vi "FestoCPX.Station.TowerHorn.Fglb.vi"(7 "Action (get)":T1=enum."get", 8 "error in":errorcluster, 10 "Period [s]":dbl) -> (0 "error out":errorcluster, 2 "Done?":bool)   [LabVIEW 2016]
uses:
  FestoCPX.Station.TowerHorn.Fglb.Action.ctl
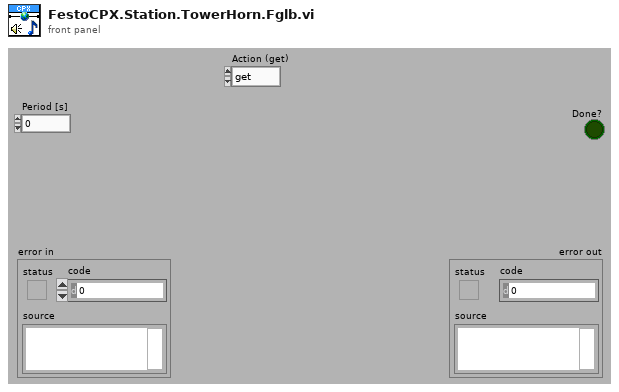
[diagram p1: front panel]
types:
  T1 = typedef "FestoCPX.Station.TowerHorn.Fglb.Action.ctl" = enum16{"init", "set", "get"}
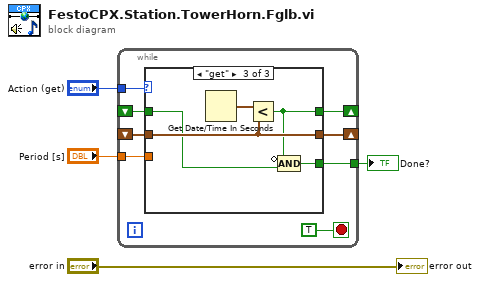
[diagram p0: block diagram]
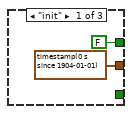
[diagram p2: hidden frame]
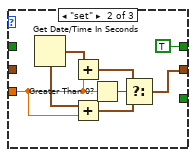
[diagram p3: hidden frame]
diagram:
  n1 = while {
    tunnel: "Action (get)" -> [w11]
    tunnel: "Period [s]" -> [w10]
    shift-right: [w9] -> _
    shift-left: _ -> [w8]
    shift-right: [w7] -> _
    shift-left: _ -> [w6]
    tunnel: [w5] -> w1
    stop <- TRUE stop-if-true
    n2 = case shown="\"get\"" w11 {
      tunnel: w10 -> [_ w15 _]
      tunnel: [timestamp(0 s since 1904-01-01) w18 w25] -> w9
      tunnel: w8 -> [_ _ w25]
      tunnel: [FALSE TRUE w24] -> w7
      tunnel: w6 -> [_ _ w23]
      tunnel: [_ _ w22] -> w5
      frame "init" {
      }
      frame "set" {
        n3 = Get Date/Time In Seconds() -> (seconds since 1Jan1904=w17:timestamp)
        n4 = Add(x=w17, y=w15) -> (x+y=w19:timestamp)
        n5 = Add(x=w17, y=w15) -> (x+y=w16:timestamp)
        n6 = Greater Than 0?(x=w15) -> (x > 0?=w20:bool)
        n7 = Select(t=w19, s=w20, f=w16) -> (s? t:f=w18:timestamp)
      }
      frame "get" {
        n8 = Get Date/Time In Seconds() -> (seconds since 1Jan1904=w26:timestamp)
        n9 = Less?(x=w26, y=w25) -> (x < y?=w24:bool)
        n10 = Compound Arithmetic op=AND(invert w24, w23) -> (w22:bool)
      }
    }
  }
  "Done?" <- w1
  "error out" <- "error in"
